vi "Restarts Loop.vi"(11 "FPGA Ref":T1) -> ()   [LabVIEW 2019]
uses:
  Controls/FPGA_Reference.ctl
  <vilib>/Platform/TimedLoop/XDataNode/timing_clust.ctl
  <vilib>/Platform/TimedLoop/XDataNode/nitl_modes.ctl
  <vilib>/Platform/TimedLoop/XDataNode/wakeup.ctl
  Type Defs/Crash File Mode.ctl
  Type Defs/Crash File State.ctl
  <vilib>/Utility/error.llb/Error Cluster From Error Code.vi
  <vilib>/rvi/errors/niLvFpgaAdjustHostInterfaceError.vi
  <vilib>/Platform/TimedLoop/XDataNode/XDataNode.xnode
  <vilib>/rvi/interface/nirviReadWriteControl/nirviReadWriteControl.xnode
  FPGA Bitfiles/TI sbRIO Main (FPGA, 9627).lvbitx
  <vilib>/Platform/TimedLoop/XDataNode/XDNodeRunTimeDep.lvlib
  NiFpgaLv.dll
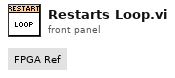
[diagram p1: front panel]
types:
  T1 = typedef "FPGA_Reference.ctl" = refnum<k20>
  T2 = typedef "XDNodeRunTimeDep.lvlib/timing_clust.ctl" = cluster{"Expected End [f-1]":u64, "Actual End [f-1]":u64, "Finished Late? [f-1]":bool, "Expected End [i-1]":u64, "Actual End [i-1]":u64, "Finished Late? [i-1]":bool, "Expected Start [i]":u64, "Actual Start [i]":u64, "Expected Start [f]":u64, "Actual Start [f]":u64, "Source Name":string, "Structure Name":string, "Period":i64, "Deadline":i64, "Offset":i64, "Start":i64, "Priority":i32, "Timeout":i32, "Mode":T3, "Wakeup Reason":T4, "Error":errorcluster, "Source Type":string, "Secondary Source Type":string, "Global End Time":u64, "Global Start Time":u64, "Frame Duration":u64, "Iteration Duration":u64, "Assigned CPU":i32, "I/O Scan Engine Mode":u32}
  T3 = typedef "XDNodeRunTimeDep.lvlib/nitl_modes.ctl" = enum32{"No Change", "Process missed periods, maintain original phase", "Discard missed periods, maintain original phase", "Process missed periods, ignore original phase", "Discard missed periods, ignore original phase"}
  T4 = typedef "XDNodeRunTimeDep.lvlib/wakeup.ctl" = enum32{"Normal", "Aborted", "Asynchronous wakeup", "Timing source error", "Timed loop error", "Timeout"}
  T5 = typedef "Crash File Mode.ctl" = enum16{"Pump 1 Write", "Pump 2 Write", "Pump 3 Write", "Pump 4 Write", "Pump 5 Write", "Pump 6 Write", "Read All", "Init"}
  T6 = typedef "Crash File State.ctl" = enum16{"Idle", "Alarm Triggered", "Alarm Latched"}
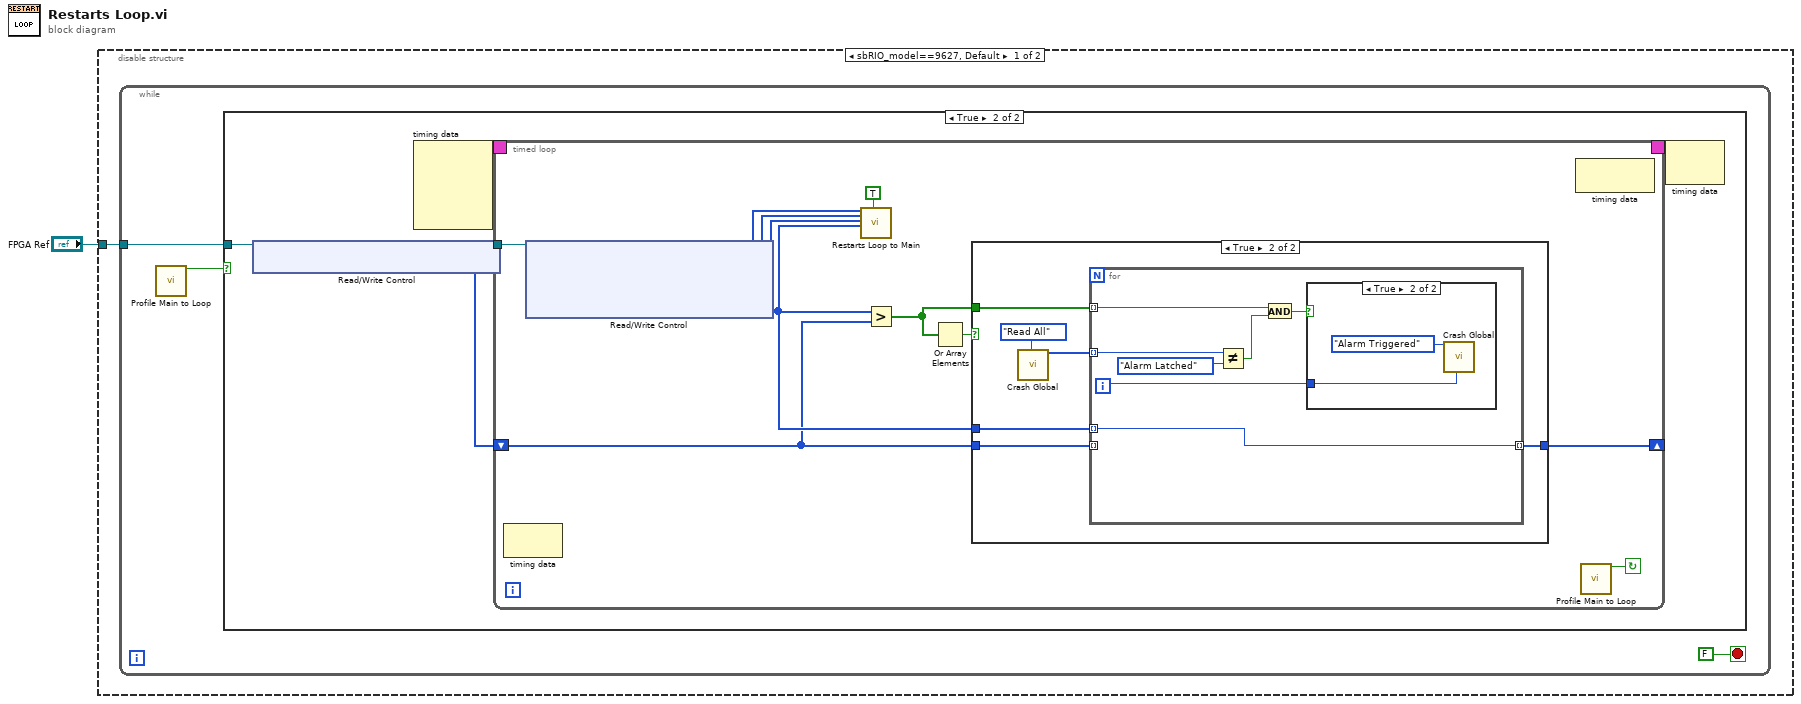
[diagram p0: block diagram]
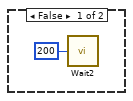
[diagram p2: hidden frame]
diagram:
  n1 = disable-structure shown="sbRIO_model==9627, Default" {
    disable-tunnel: "FPGA Ref" -> [w2 _]
    frame condition #0 (active) {
      n2 = while {
        tunnel: w2 -> [w3]
        stop <- FALSE stop-if-true
        n3 = call "Profile Main to Loop.vi"() -> ("Run Profile OUT"=w4:bool)  [unwired: 14 in, 5 out]
        n4 = case shown="True" w4 {
          tunnel: w3 -> [_ w9]
          frame False {
            n5 = call "Wait2"("Count(mSec)"=u32 200) -> ()  [unwired: 1 out]
          }
          frame True {
            n6 = xnode "Read/Write Control"("FPGA VI Reference In"=w9) -> ("FPGA VI Reference Out"=w8:T1, "Restarts"=w7:i32[])  [unwired: 1 in, 1 out]
            n7 = node-c288() -> (w11:T2)  [unwired: 4 in]
            n8 = timed-loop {
              tunnel: w8 -> [w21]
              timing: w11 -> [_]
              timing-out: [_] -> w10
              shift-right: [w15] -> _
              shift-left: w7 -> [w13]
              stop <- w22 continue-if-true
              n9 = node-c288() -> ()  [unwired: 1 in, 1 out]
              n10 = xnode "Read/Write Control"("FPGA VI Reference In"=w21) -> ("Actual Pump Starts"=w18:u32[], "Cmd Pump Starts"=w17:u32[], "Pump No Starts"=w16:u32[], "Restarts"=w14:i32[])  [unwired: 1 in, 2 out]
              n11 = call "Restarts Loop to Main.vi"("Actual Pump Starts"=w18, "Cmd Pump Starts"=w17, "Pump No Starts"=w16, "Restarts"=w14, "Write (F)"=TRUE) -> ()  [unwired: 10 in, 5 out]
              n12 = Greater?(x=w14, y=w13) -> (0:w12:bool[])
              n13 = Or Array Elements(Boolean array=w12) -> (logical OR=w20:bool)
              n14 = case shown="True" w20 {
                tunnel: w12 -> [_ w31]
                tunnel: w13 -> [w25 w28]
                tunnel: w14 -> [_ w27]
                tunnel: [w25 w26] -> w15
                frame False {
                }
                frame True {
                  n15 = call "Crash Global.vi"("Mode"=Crash_File_Mode."Read All") -> ("Crash File States"=w29:T6[])  [unwired: 17 in, 1 out]
                  n16 = for {
                    tunnel: w31 -> [w35] mode=indexing
                    tunnel: w29 -> [w37] mode=indexing
                    tunnel: w28 -> [_] mode=indexing
                    tunnel: w27 -> [w32] mode=indexing
                    tunnel: [w32] -> w26 mode=indexing
                    i -> [w38]
                    n17 = Not Equal?(x=w37, y=Crash_File_State."Alarm Latched") -> (x != y?=w34:bool)
                    n18 = And(x=w35, y=w34) -> (x .and. y?=w33:bool)
                    n19 = case shown="True" w33 {
                      tunnel: w38 -> [_ w39]
                      frame False {
                      }
                      frame True {
                        n20 = call "Crash Global.vi"("Crash State IN"=Crash_File_State."Alarm Triggered", "Mode"=w39) -> ()  [unwired: 16 in, 2 out]
                      }
                    }
                  }
                }
              }
              n21 = node-c288() -> ()  [unwired: 1 in, 1 out]
              n22 = call "Profile Main to Loop.vi"() -> ("Run Profile OUT"=w22:bool)  [unwired: 14 in, 5 out]
            }
            n23 = node-c288(w10) -> ()  [unwired: 1 out]
          }
        }
      }
    }
    frame condition #1 {
    }
  }
